vi "Main.vi"(11 "Module Admin":refnum<class "Delacor_lib_QMH_Cloneable Module Admin.lvclass">) -> ()   [LabVIEW 2025, in "Power Supply.lvlib"]
doc: "This template is based off of the Queued Message Handler design pattern and the Queued Message Handler project template that ships with LabVIEW.\n\nThe main difference is that the queue is private to this module and communication between modules is performed via Broadcast and Request events.\n\nRequest events are wrapped in public API methods and are handled in the Event Handling Loop (EHL) of this VI. Any module can register for Broadcast events sent by this module. The EHL generates messages based on user interface actions.\n\nThe Message Handling Loop (MHL) processes messages generated by the EHL, or by other messages. The messages are string values, so new messages can be added easily to the Message Cases case structure in the MHL. Each message cluster can also provide an optional value for Message Data, which is a variant that can be converted to whatever message-specific data is required.\n_____\nBased on DQMH Dev Tools: Project Template 7.1.2.1547."
uses:
  Power Supply.lvlib
  <vilib>/Delacor/Delacor QMH/Libraries/Message Queue_class/Delacor_lib_QMH_Message Queue.lvclass
  Module Data--cluster.ctl
  <vilib>/Utility/miscctls.llb/LVPointTypeDef.ctl
  <vilib>/Delacor/Delacor QMH/Libraries/Message Queue_class/Delacor_lib_QMH_Enqueue Message (Single).vi
  Stop Argument--cluster.ctl
  <vilib>/Delacor/Delacor QMH/Libraries/Cloneable Module Admin_class/Delacor_lib_QMH_Cloneable Module Admin.lvclass
  select child (Reply Payload)--cluster.ctl
  Classes/hardware-selection.ctl
  select child Argument--cluster.ctl
  Classes/generic-power-supply/generic-power-supply.lvclass
  Classes/PSP-603/PSP-603.lvclass
  read config (Reply Payload)--cluster.ctl
  read config Argument--cluster.ctl
  init device (Reply Payload)--cluster.ctl
  init device Argument--cluster.ctl
  close (Reply Payload)--cluster.ctl
  close Argument--cluster.ctl
  output (Reply Payload)--cluster.ctl
  output Argument--cluster.ctl
  set voltage (Reply Payload)--cluster.ctl
  set voltage Argument--cluster.ctl
  set current (Reply Payload)--cluster.ctl
  set current Argument--cluster.ctl
  Controls/Numeric Current.ctl
  read current (Reply Payload)--cluster.ctl
  read current Argument--cluster.ctl
  Controls/Numeric Voltage.ctl
  read voltage (Reply Payload)--cluster.ctl
  read voltage Argument--cluster.ctl
  read state (Reply Payload)--cluster.ctl
  read state Argument--cluster.ctl
  set all outputs (Reply Payload)--cluster.ctl
  set all outputs Argument--cluster.ctl
  C:/Users/grove/Desktop/LabVIEW/Git/atp-station/Libraries/Power Supply/Classes/generic-power-supply/generic-power-supply.lvclass
  C:/Users/grove/Desktop/LabVIEW/Git/atp-station/Libraries/Power Supply/Classes/PSP-603/PSP-603.lvclass
panel:
  out "error out":errorcluster
  out "Status":string
  in  "Simulate EHL Error":bool
  in  "Simulate MHL Error":bool
  # "Other processes communicate with this Module via its Public API (wrappers for its Request Events).\n\nThis Module communicates with other processes via its Broadcast Events.\nAny process that wants to receive these messages can register for this module's Broadcast events."
  # "This template is for the DQMH framework. See the block diagram for more information on how to use this template."
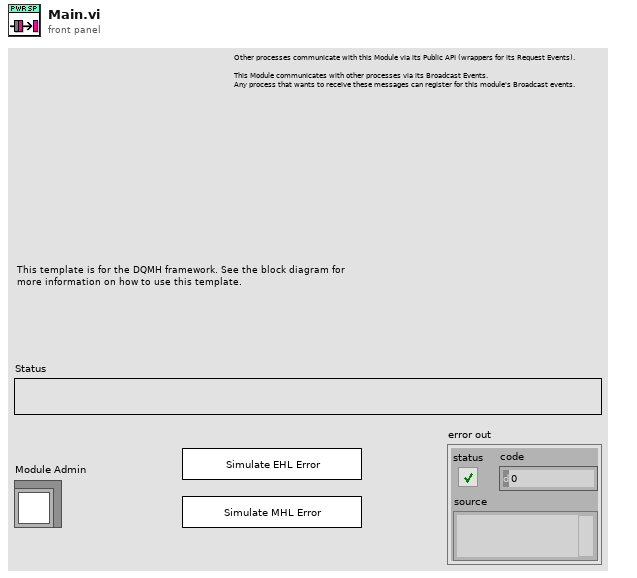
[diagram p1: front panel]
types:
  T1 = typedef "Power Supply.lvlib/Request Events--cluster.ctl" = cluster{"Stop Module":refnum<user-event>, "Show Panel":refnum<user-event>, "Hide Panel":refnum<user-event>, "Show Diagram":refnum<user-event>, "Get Module Execution Status":refnum<user-event>, "select child":refnum<user-event>, "read config":refnum<user-event>, "init device":refnum<user-event>, "close":refnum<user-event>, "output":refnum<user-event>, "set voltage":refnum<user-event>, "set current":refnum<user-event>, "read current":refnum<user-event>, "read voltage":refnum<user-event>, "read state":refnum<user-event>, "set all outputs":refnum<user-event>}
  T2 = typedef "Power Supply.lvlib/Module Data--cluster.ctl" = cluster{"Status":string, "Power Supply Object":refnum<class "generic-power-supply.lvclass">}
  T3 = enum32{"invalid lock state", "Not Locked", "Locked (No Password)", "Password-protected"}
  T4 = typedef "Power Supply.lvlib/Stop Argument--cluster.ctl" = cluster{"Module ID":i32, "Origin":string, "Exit via Stop Module Req?":bool, "Wait for Module to stop?":bool}
  T5 = typedef "Power Supply.lvlib/select child Argument--cluster.ctl" = cluster{"Module ID":i32, "Enum":T6, "Wait Notifier":refnum<notifier>, "wait for reply":bool}
  T6 = typedef "hardware-selection.ctl" = enum16{"Parent", "Simulation", "PSP-603"}
  T7 = typedef "Power Supply.lvlib/read config Argument--cluster.ctl" = cluster{"Module ID":i32, "config json file":path, "Wait Notifier":refnum<notifier>, "wait for reply":bool}
  T8 = typedef "Power Supply.lvlib/init device Argument--cluster.ctl" = cluster{"Module ID":i32, "Variant":variant, "Wait Notifier":refnum<notifier>, "wait for reply":bool}
  T9 = typedef "Power Supply.lvlib/close Argument--cluster.ctl" = cluster{"Module ID":i32, "Wait Notifier":refnum<notifier>, "wait for reply":bool}
  T10 = typedef "Power Supply.lvlib/output Argument--cluster.ctl" = cluster{"Module ID":i32, "Output On/Off":bool, "Wait Notifier":refnum<notifier>, "wait for reply":bool}
  T11 = typedef "Power Supply.lvlib/set voltage Argument--cluster.ctl" = cluster{"Module ID":i32, "Output Voltage":dbl, "Wait Notifier":refnum<notifier>, "wait for reply":bool}
  T12 = typedef "Power Supply.lvlib/set current Argument--cluster.ctl" = cluster{"Module ID":i32, "Output Current":dbl, "Wait Notifier":refnum<notifier>, "wait for reply":bool}
  T13 = typedef "Power Supply.lvlib/read current Argument--cluster.ctl" = cluster{"Module ID":i32, "Wait Notifier":refnum<notifier>, "wait for reply":bool}
  T14 = typedef "Power Supply.lvlib/read voltage Argument--cluster.ctl" = cluster{"Module ID":i32, "Wait Notifier":refnum<notifier>, "wait for reply":bool}
  T15 = typedef "Power Supply.lvlib/read state Argument--cluster.ctl" = cluster{"Module ID":i32, "Wait Notifier":refnum<notifier>, "wait for reply":bool}
  T16 = typedef "Power Supply.lvlib/set all outputs Argument--cluster.ctl" = cluster{"Module ID":i32, "Voltage":dbl, "Current":dbl, "Output On/Off":bool, "Wait Notifier":refnum<notifier>, "wait for reply":bool}
  T17 = typedef "LVPointTypeDef.ctl" = cluster{"Horizontal":i16, "Vertical":i16}
  T18 = enum32{"Invalid", "Standard", "Closed", "Hidden", "Minimized", "Maximized"}
  T19 = typedef "Power Supply.lvlib/select child (Reply Payload)--cluster.ctl" = cluster{"Module ID":i32, "error":errorcluster}
  T20 = typedef "Power Supply.lvlib/read config (Reply Payload)--cluster.ctl" = cluster{"Module ID":i32, "error":errorcluster}
  T21 = typedef "Power Supply.lvlib/init device (Reply Payload)--cluster.ctl" = cluster{"Module ID":i32, "error":errorcluster}
  T22 = typedef "Power Supply.lvlib/close (Reply Payload)--cluster.ctl" = cluster{"Module ID":i32, "error":errorcluster}
  T23 = typedef "Power Supply.lvlib/output (Reply Payload)--cluster.ctl" = cluster{"Module ID":i32, "error":errorcluster}
  T24 = typedef "Power Supply.lvlib/set voltage (Reply Payload)--cluster.ctl" = cluster{"Module ID":i32, "error":errorcluster}
  T25 = typedef "Power Supply.lvlib/set current (Reply Payload)--cluster.ctl" = cluster{"Module ID":i32, "error":errorcluster}
  T26 = typedef "Power Supply.lvlib/read current (Reply Payload)--cluster.ctl" = cluster{"Module ID":i32, "Amps":T27, "error":errorcluster}
  T27 = typedef "Numeric Current.ctl" = dbl
  T28 = typedef "Power Supply.lvlib/read voltage (Reply Payload)--cluster.ctl" = cluster{"Module ID":i32, "Volts":T29, "error":errorcluster}
  T29 = typedef "Numeric Voltage.ctl" = dbl
  T30 = typedef "Power Supply.lvlib/read state (Reply Payload)--cluster.ctl" = cluster{"Module ID":i32, "Variant":variant, "error":errorcluster}
  T31 = typedef "Power Supply.lvlib/set all outputs (Reply Payload)--cluster.ctl" = cluster{"Module ID":i32, "error":errorcluster}
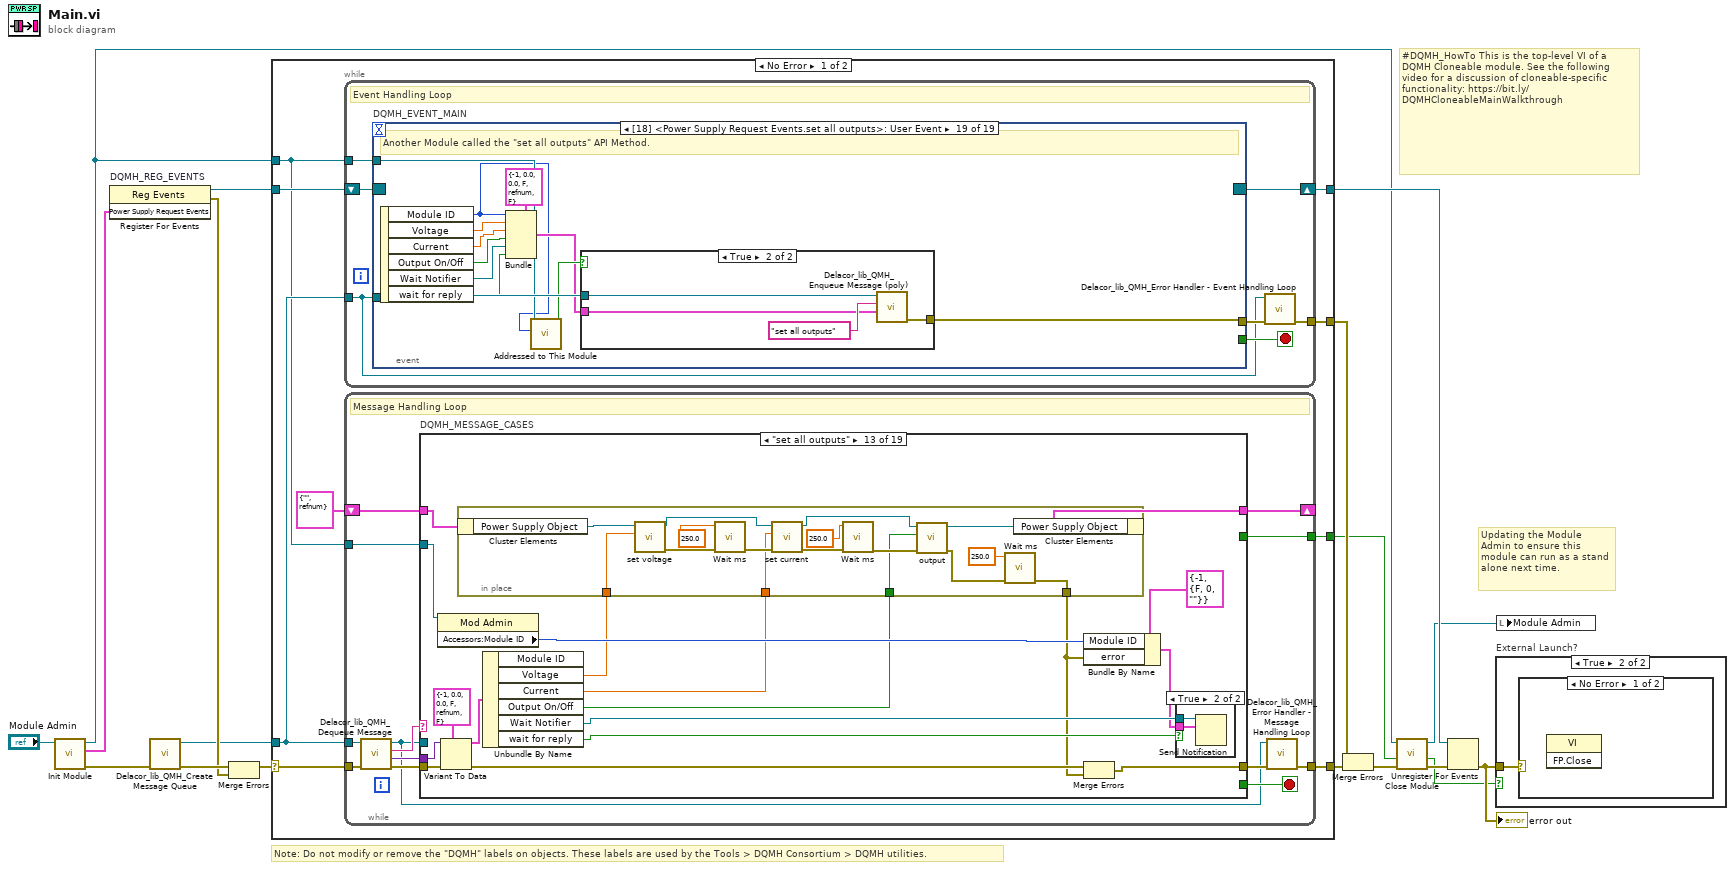
[diagram p0: block diagram]
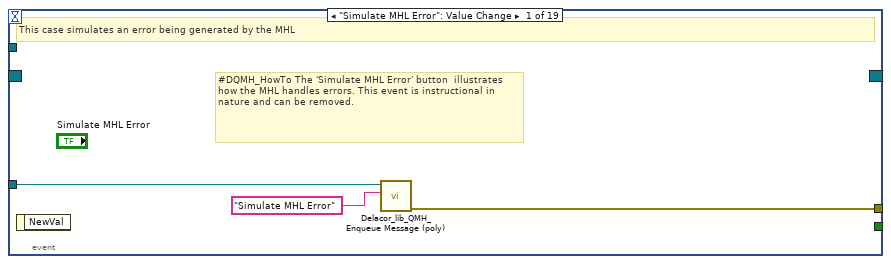
[diagram p2: hidden frame]
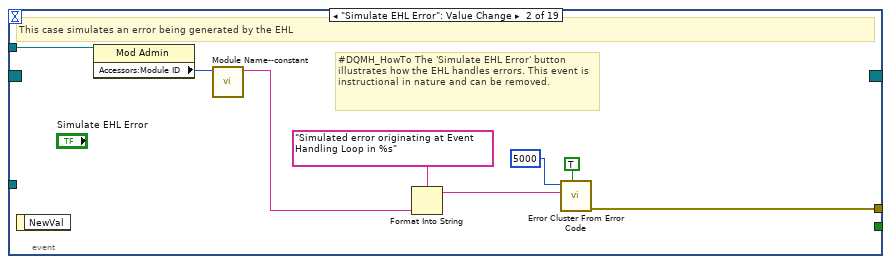
[diagram p3: hidden frame]
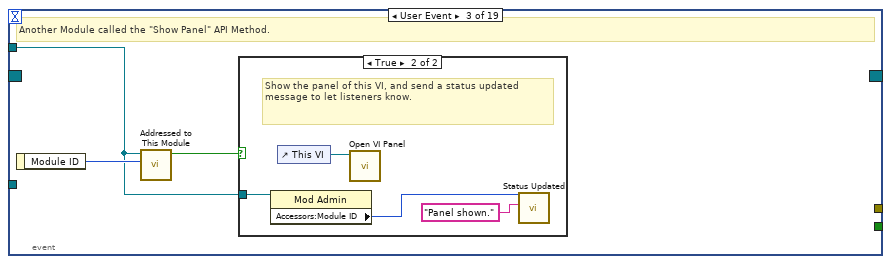
[diagram p4: hidden frame]
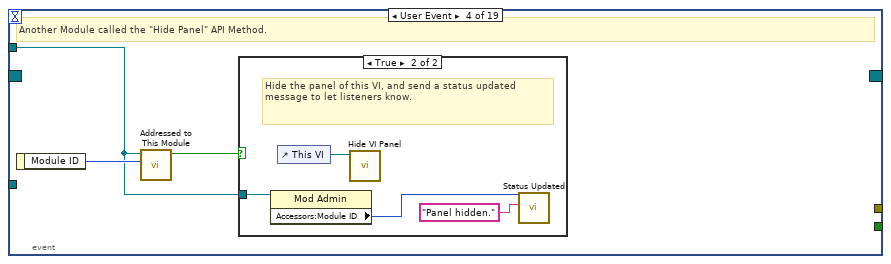
[diagram p6: hidden frame]
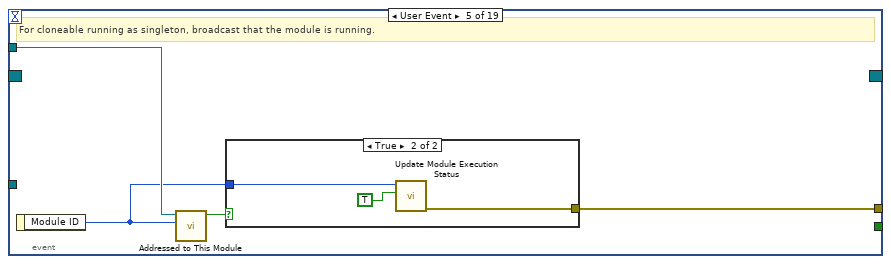
[diagram p8: hidden frame]
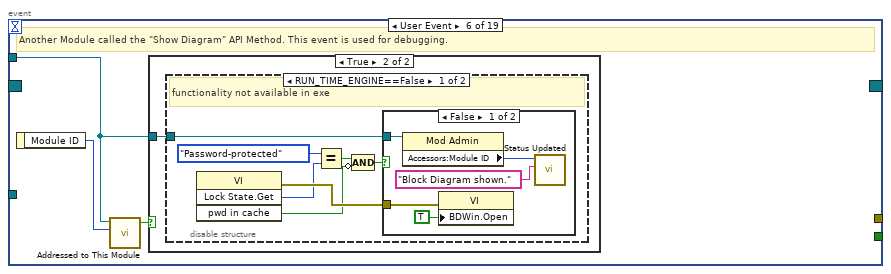
[diagram p10: hidden frame]
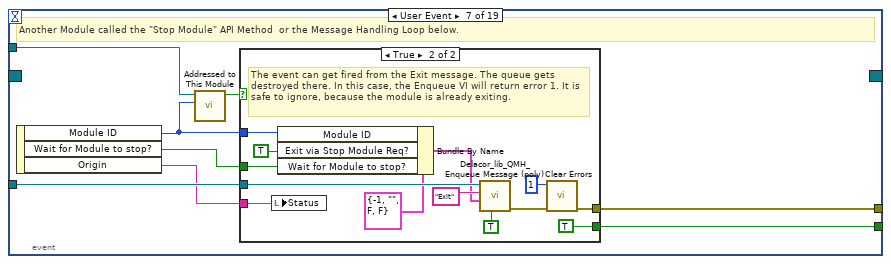
[diagram p14: hidden frame]
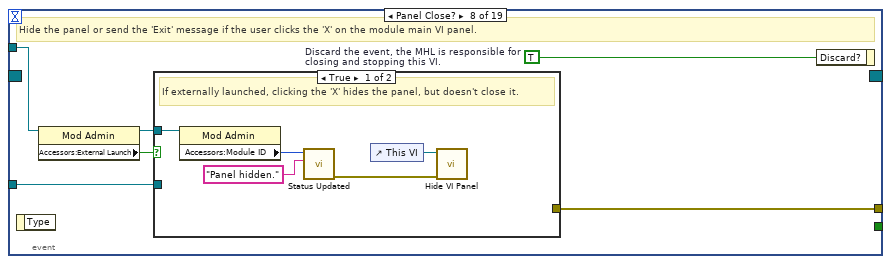
[diagram p16: hidden frame]
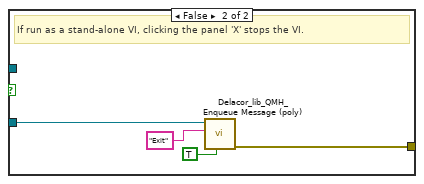
[diagram p17: hidden frame]
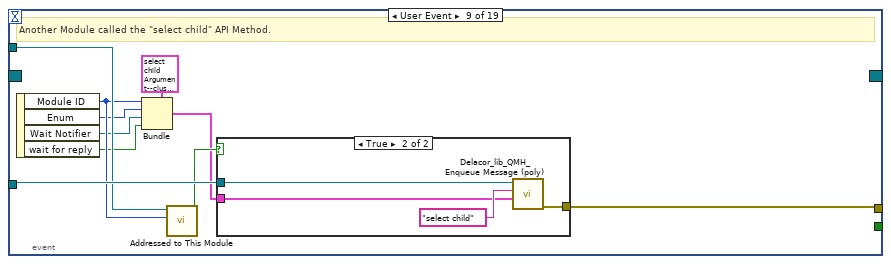
[diagram p18: hidden frame]
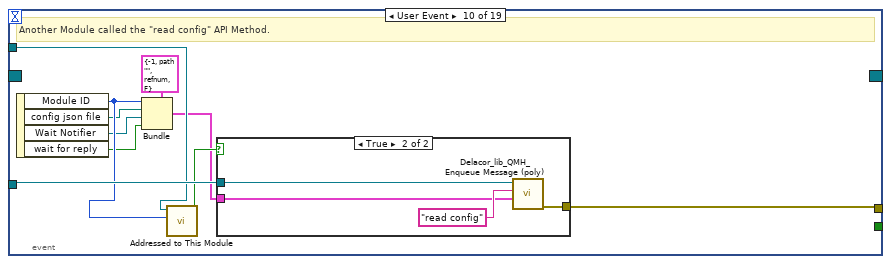
[diagram p20: hidden frame]
diagram:
  # "#DQMH_HowTo This is the top-level VI of a DQMH Cloneable module. See the following video for a discussion of cloneable-specific functionality: https://bit.ly/DQMHCloneableMainWalkthrough"
  # "Note: Do not modify or remove the \"DQMH\" labels on objects. These labels are used by the Tools > DQMH Consortium > DQMH utilities."
  # "Updating the Module Admin to ensure this module can run as a stand alone next time."
  n1 = call "Init Module.vi"("Cloneable Module Admin in"="Module Admin") -> ("error out"=w15:errorcluster, "Power Supply Request Events"=w7:T1, "Cloneable Module Admin out"=w4:refnum<class "Delacor_lib_QMH_Cloneable Module Admin.lvclass">)  [unwired: 8 in]
  n2 = register-events "DQMH_REG_EVENTS"(w7) -> (reference out=w8:refnum<event-registration>, error out=w10:errorcluster)  [unwired: 2 in]
  n3 = call <vilib>:"Delacor_lib_QMH_Create Message Queue.vi"("error in"=w15) -> ("error out"=w12:errorcluster, "Message Queue"=w6:refnum<class "Delacor_lib_QMH_Message Queue.lvclass">)  [unwired: 9 in]
  n4 = Merge Errors(w12, w10) -> (w11:errorcluster)
  n5 = case shown="No Error" w11 {
    selector: w11 -> [w25 w634]
    tunnel: [w27 w633] -> w16
    tunnel: [w24 w632] -> w9
    tunnel: w8 -> [w22 w632]
    tunnel: w6 -> [w21 w625]
    tunnel: [w26 _] -> w17
    tunnel: w4 -> [w20 w628]
    tunnel: [w19 _] -> w2
    frame No Error {
      n6 = while {
        tunnel: w21 -> [w28]
        shift-right: [w31] -> w24
        shift-left: w22 -> [w32]
        tunnel: [w33] -> w26
        tunnel: w20 -> [w29]
        stop <- w30 stop-if-true
        # "Event Handling Loop"
        n7 = event "DQMH_EVENT_MAIN" shown="[18] <Power Supply Request Events.set all outputs>: User Event" {
          selector: w32 -> [_ _ _ _ _ _ _ _ _ _ _ _ _ _ _ _ _ _ _]
          dyn-events: [_ _ _ _ _ _ _ _ _ _ _ _ _ _ _ _ _ _ _] -> w31
          timeout: _ -> [_ _ _ _ _ _ _ _ _ _ _ _ _ _ _ _ _ _ _]
          tunnel: [_ _ _ _ _ _ w86 _ _ _ _ _ _ _ _ _ _ _ _] -> w30
          tunnel: w28 -> [w36 _ _ _ _ _ w89 w106 w128 w142 w156 w169 w183 w197 w211 w224 w237 w250 w266]
          tunnel: [w37 w45 _ _ w63 _ w90 w109 w119 w133 w147 w161 w174 w188 w202 w216 w229 w242 w255] -> w34
          tunnel: w29 -> [_ w44 w46 w53 w61 w67 w88 w107 w126 w140 w154 w167 w181 w195 w209 w222 w235 w248 w264]
          event "Simulate MHL Error": Value Change {
            # "#DQMH_HowTo The 'Simulate MHL Error' button  illustrates how the MHL handles errors. This event is instructional in nature and can be removed."
            # "This case simulates an error being generated by the MHL"
            n8 = event-data() -> ()  [unwired: 1 in, 1 out]
            n9 = call-poly <vilib>:"Delacor_lib_QMH_Enqueue Message (poly).vi"("Message"="Simulate MHL Error", "Message Queue in"=w36) -> ("error out"=w37:errorcluster)  [unwired: 8 in, 1 out]
          }
          event "Simulate EHL Error": Value Change {
            # "#DQMH_HowTo The 'Simulate EHL Error' button  illustrates how the EHL handles errors. This event is instructional in nature and can be removed."
            # "This case simulates an error being generated by the EHL"
            n10 = event-data() -> ()  [unwired: 1 in, 1 out]
            n11 = property on="Property Node" class="Mod Admin"(reference=w44) -> ("Accessors:Module ID"=w43:i32)  [unwired: 1 in, 2 out]
            n12 = call "Module Name--constant.vi"("Module ID"=w43) -> ("Module Name"=w38:string)  [unwired: 10 in]
            n13 = Format Into String(format string="Simulated error originating at Event Handling Loop in %s", w38) -> (resulting string=w41:string)  [unwired: 2 in, 1 out]
            n14 = call <vilib>:"Error Cluster From Error Code.vi"("show call chain? (False)"=TRUE, "error message (\"\")"=w41, "error code (0)"=5000) -> ("error out"=w45:errorcluster)  [unwired: 6 in]
          }
          event User Event {
            # "Another Module called the \"Show Panel\" API Method."
            n15 = event-data() -> ("Module ID"=w47:i32)  [unwired: 1 in]
            n16 = call "Addressed to This Module.vi"("Module ID from Argument"=w47, "Module Admin"=w46) -> ("Addressed to this instance?"=w48:bool)  [unwired: 8 in, 1 out]
            n17 = case shown="True" w48 {
              tunnel: w46 -> [_ w50]
              frame False {
              }
              frame True {
                # "Show the panel of this VI, and send a status updated message to let listeners know."
                n18 = property on="Property Node" class="Mod Admin"(reference=w50) -> ("Accessors:Module ID"=w49:i32)  [unwired: 1 in, 2 out]
                n19 = control-ref of="This VI"() -> (w52:refnum<vi>)
                n20 = call "Open VI Panel.vi"("VI"=w52) -> ()  [unwired: 10 in, 1 out]
                n21 = call "Status Updated.vi"("Status"="Panel shown." ("format string"), "Module ID"=w49) -> ()  [unwired: 9 in, 1 out]
              }
            }
          }
          event User Event {
            # "Another Module called the \"Hide Panel\" API Method."
            n22 = event-data() -> ("Module ID"=w54:i32)  [unwired: 1 in]
            n23 = call "Addressed to This Module.vi"("Module ID from Argument"=w54, "Module Admin"=w53) -> ("Addressed to this instance?"=w55:bool)  [unwired: 8 in, 1 out]
            n24 = case shown="True" w55 {
              tunnel: w53 -> [_ w57]
              frame False {
              }
              frame True {
                # "Hide the panel of this VI, and send a status updated message to let listeners know."
                n25 = property on="Property Node" class="Mod Admin"(reference=w57) -> ("Accessors:Module ID"=w56:i32)  [unwired: 1 in, 2 out]
                n26 = control-ref of="This VI"() -> (w59:refnum<vi>)
                n27 = call "Hide VI Panel.vi"("VI"=w59) -> ()  [unwired: 10 in, 1 out]
                n28 = call "Status Updated.vi"("Status"="Panel hidden." ("format string"), "Module ID"=w56) -> ()  [unwired: 9 in, 1 out]
              }
            }
          }
          event User Event {
            # "For cloneable running as singleton, broadcast that the module is running."
            n29 = event-data() -> ("Module ID"=w60:i32)  [unwired: 1 in]
            n30 = call "Addressed to This Module.vi"("Module ID from Argument"=w60, "Module Admin"=w61) -> ("Addressed to this instance?"=w62:bool)  [unwired: 8 in, 1 out]
            n31 = case shown="True" w62 {
              tunnel: [_ w66] -> w63
              tunnel: w60 -> [_ w65]
              frame False {
              }
              frame True {
                n32 = call "Update Module Execution Status.vi"("Running?"=TRUE, "Module ID"=w65) -> ("error out"=w66:errorcluster)  [unwired: 9 in]
              }
            }
          }
          event User Event {
            # "Another Module called the \"Show Diagram\" API Method. This event is used for debugging."
            n33 = event-data() -> ("Module ID"=w68:i32)  [unwired: 1 in]
            n34 = call "Addressed to This Module.vi"("Module ID from Argument"=w68, "Module Admin"=w67) -> ("Addressed to this instance?"=w69:bool)  [unwired: 8 in, 1 out]
            n35 = case shown="True" w69 {
              tunnel: w67 -> [_ w70]
              frame False {
              }
              frame True {
                n36 = disable-structure shown="RUN_TIME_ENGINE==False" {
                  disable-tunnel: w70 -> [w71 _]
                  frame condition #0 (active) {
                    # "functionality not available in exe"
                    n37 = invoke on="Invoke Node" class="VI" method="Lock State.Get"() -> (error out=w77:errorcluster, "Get Lock State"=w76:T3, "pwd in cache"=w73:bool)  [unwired: 4 in, 1 out]
                    n38 = Equal?(x=T3."Password-protected", y=w76) -> (x = y?=w74:bool)
                    n39 = Compound Arithmetic op=AND(w74, invert w73) -> (w72:bool)
                    n40 = case shown="False" w72 {
                      tunnel: w77 -> [w82 _]
                      tunnel: w71 -> [w79 _]
                      frame False {
                        n41 = property on="Property Node" class="Mod Admin"(reference=w79) -> ("Accessors:Module ID"=w78:i32)  [unwired: 1 in, 2 out]
                        n42 = property on="Property Node" class="VI"(error in=w82, "BDWin.Open"=TRUE ("Block Diagram Window:Open")) -> ()  [unwired: 1 in, 2 out]
                        n43 = call "Status Updated.vi"("Status"="Block Diagram shown." ("format string"), "Module ID"=w78) -> ()  [unwired: 9 in, 1 out]
                      }
                      frame True {
                        # "Password-protected VI, and the password is not in the cache. Do not show the diagram."
                      }
                    }
                  }
                  frame condition #1 {
                  }
                }
              }
            }
          }
          event User Event {
            # "Another Module called the \"Stop Module\" API Method  or the Message Handling Loop below."
            n44 = event-data() -> ("Module ID"=w84:i32, "Wait for Module to stop?"=w85:bool, "Origin"=w83:string)  [unwired: 1 in]
            n45 = call "Addressed to This Module.vi"("Module ID from Argument"=w84, "Module Admin"=w88) -> ("Addressed to this instance?"=w87:bool)  [unwired: 8 in, 1 out]
            n46 = case shown="True" w87 {
              tunnel: [_ w102] -> w90
              tunnel: w89 -> [_ w98]
              tunnel: [_ TRUE] -> w86
              tunnel: w85 -> [_ w93]
              tunnel: w84 -> [_ w95]
              tunnel: w83 -> [_ w91]
              frame False {
              }
              frame True {
                # "The event can get fired from the Exit message. The queue gets destroyed there. In this case, the Enqueue VI will return error 1. It is safe to ignore, because the module is already exiting."
                n47 = local write "Status"(w91) -> ()
                n48 = Bundle By Name(cluster=T4 {"Module ID"=-1, "Origin"="", "Exit via Stop Module Req?"=FALSE, "Wait for Module to stop?"=FALSE} ("Stop Argument"), "Module ID"=w95, "Exit via Stop Module Req?"=TRUE, "Wait for Module to stop?"=w93) -> (w92:T4)
                n49 = call-poly <vilib>:"Delacor_lib_QMH_Enqueue Message (poly).vi"("Priority Message? (F)"=TRUE, "Message Data"=w92, "Message"="Exit", "Message Queue in"=w98) -> ("error out"=w103:errorcluster)  [unwired: 6 in, 1 out]
                n50 = call <vilib>:"Clear Errors.vi"("error in (no error)"=w103, "specific error code to clear (0: all)"=1) -> ("error out"=w102:errorcluster)  [unwired: 4 in, 1 out]
              }
            }
          }
          event Panel Close? {
            w108 = TRUE  # Discard the event, the MHL is responsible for closing and stopping this VI.
            # "Hide the panel or send the 'Exit' message if the user clicks the 'X' on the module main VI panel."
            n51 = event-data() -> ()  [unwired: 1 in, 1 out]
            n52 = property on="Property Node" class="Mod Admin"(reference=w107) -> (reference out=w104:refnum<class "Delacor_lib_QMH_Cloneable Module Admin.lvclass">, "Accessors:External Launch"=w105:bool)  [unwired: 1 in, 1 out]
            n53 = case shown="True" w105 {
              tunnel: w106 -> [_ w117]
              tunnel: [_ w118] -> w109
              tunnel: w104 -> [w112 _]
              frame True {
                # "If externally launched, clicking the 'X' hides the panel, but doesn't close it."
                n54 = property on="Property Node" class="Mod Admin"(reference=w112) -> ("Accessors:Module ID"=w111:i32)  [unwired: 1 in, 2 out]
                n55 = call "Status Updated.vi"("Status"="Panel hidden." ("format string"), "Module ID"=w111) -> ("error out"=w110:errorcluster)  [unwired: 9 in]
                n56 = control-ref of="This VI"() -> (w114:refnum<vi>)
                n57 = call "Hide VI Panel.vi"("error in"=w110, "VI"=w114) -> ()  [unwired: 9 in, 1 out]
              }
              frame False {
                # "If run as a stand-alone VI, clicking the panel 'X' stops the VI."
                n58 = call-poly <vilib>:"Delacor_lib_QMH_Enqueue Message (poly).vi"("Priority Message? (F)"=TRUE, "Message"="Exit", "Message Queue in"=w117) -> ("error out"=w118:errorcluster)  [unwired: 7 in, 1 out]
              }
            }
            n59 = event-data ("Event Filter Node")("Discard?"=w108) -> ()  [unwired: 1 in, 1 out]
          }
          event User Event {
            # "Another Module called the \"select child\" API Method."
            n60 = event-data() -> ("Module ID"=w123:i32, "Enum"=w122:T6, "Wait Notifier"=w121:refnum<notifier>, "wait for reply"=w120:bool)  [unwired: 1 in]
            n61 = Bundle(cluster=T5 {"Module ID"=-1, "Enum"=enum."PSP-603", "Wait Notifier"=refnum, "wait for reply"=FALSE} ("select child Argument"), "Module ID"=w123, "Enum"=w122, "Wait Notifier"=w121, "wait for reply"=w120) -> (w124:T5)
            n62 = call "Addressed to This Module.vi"("Module ID from Argument"=w123, "Module Admin"=w126) -> ("Addressed to this instance?"=w127:bool)  [unwired: 8 in, 1 out]
            n63 = case shown="True" w127 {
              tunnel: w128 -> [_ w132]
              tunnel: w124 -> [_ w130]
              tunnel: [_ w129] -> w119
              frame False {
              }
              frame True {
                n64 = call-poly <vilib>:"Delacor_lib_QMH_Enqueue Message (poly).vi"("Message Data"=w130, "Message"="select child", "Message Queue in"=w132) -> ("error out"=w129:errorcluster)  [unwired: 7 in, 1 out]
              }
            }
          }
          event User Event {
            # "Another Module called the \"read config\" API Method."
            n65 = event-data() -> ("Module ID"=w137:i32, "config json file"=w136:path, "Wait Notifier"=w135:refnum<notifier>, "wait for reply"=w134:bool)  [unwired: 1 in]
            n66 = Bundle(cluster=T7 {"Module ID"=-1, "config json file"=path "", "Wait Notifier"=refnum, "wait for reply"=FALSE} ("read config Argument"), "Module ID"=w137, "config json file"=w136, "Wait Notifier"=w135, "wait for reply"=w134) -> (w138:T7)
            n67 = call "Addressed to This Module.vi"("Module ID from Argument"=w137, "Module Admin"=w140) -> ("Addressed to this instance?"=w141:bool)  [unwired: 8 in, 1 out]
            n68 = case shown="True" w141 {
              tunnel: w142 -> [_ w146]
              tunnel: w138 -> [_ w144]
              tunnel: [_ w143] -> w133
              frame False {
              }
              frame True {
                n69 = call-poly <vilib>:"Delacor_lib_QMH_Enqueue Message (poly).vi"("Message Data"=w144, "Message"="read config", "Message Queue in"=w146) -> ("error out"=w143:errorcluster)  [unwired: 7 in, 1 out]
              }
            }
          }
          event User Event {
            # "Another Module called the \"init device\" API Method."
            n70 = event-data() -> ("Module ID"=w151:i32, "Variant"=w150:variant, "Wait Notifier"=w149:refnum<notifier>, "wait for reply"=w148:bool)  [unwired: 1 in]
            n71 = Bundle(cluster=T8 {"Module ID"=-1, "Variant"=variant, "Wait Notifier"=refnum, "wait for reply"=FALSE} ("init device Argument"), "Module ID"=w151, "Variant"=w150, "Wait Notifier"=w149, "wait for reply"=w148) -> (w152:T8)
            n72 = call "Addressed to This Module.vi"("Module ID from Argument"=w151, "Module Admin"=w154) -> ("Addressed to this instance?"=w155:bool)  [unwired: 8 in, 1 out]
            n73 = case shown="True" w155 {
              tunnel: w156 -> [_ w160]
              tunnel: w152 -> [_ w158]
              tunnel: [_ w157] -> w147
              frame False {
              }
              frame True {
                n74 = call-poly <vilib>:"Delacor_lib_QMH_Enqueue Message (poly).vi"("Message Data"=w158, "Message"="init device", "Message Queue in"=w160) -> ("error out"=w157:errorcluster)  [unwired: 7 in, 1 out]
              }
            }
          }
          event User Event {
            # "Another Module called the \"close\" API Method."
            n75 = event-data() -> ("Module ID"=w164:i32, "Wait Notifier"=w163:refnum<notifier>, "wait for reply"=w162:bool)  [unwired: 1 in]
            n76 = Bundle(cluster=T9 {"Module ID"=-1, "Wait Notifier"=refnum, "wait for reply"=FALSE} ("close Argument"), "Module ID"=w164, "Wait Notifier"=w163, "wait for reply"=w162) -> (w165:T9)
            n77 = call "Addressed to This Module.vi"("Module ID from Argument"=w164, "Module Admin"=w167) -> ("Addressed to this instance?"=w168:bool)  [unwired: 8 in, 1 out]
            n78 = case shown="True" w168 {
              tunnel: w169 -> [_ w173]
              tunnel: w165 -> [_ w171]
              tunnel: [_ w170] -> w161
              frame False {
              }
              frame True {
                n79 = call-poly <vilib>:"Delacor_lib_QMH_Enqueue Message (poly).vi"("Message Data"=w171, "Message"="close", "Message Queue in"=w173) -> ("error out"=w170:errorcluster)  [unwired: 7 in, 1 out]
              }
            }
          }
          event User Event {
            # "Another Module called the \"output\" API Method."
            n80 = event-data() -> ("Module ID"=w178:i32, "Output On/Off"=w177:bool, "Wait Notifier"=w176:refnum<notifier>, "wait for reply"=w175:bool)  [unwired: 1 in]
            n81 = Bundle(cluster=T10 {"Module ID"=-1, "Output On/Off"=FALSE, "Wait Notifier"=refnum, "wait for reply"=FALSE} ("output Argument"), "Module ID"=w178, "Output On/Off"=w177, "Wait Notifier"=w176, "wait for reply"=w175) -> (w179:T10)
            n82 = call "Addressed to This Module.vi"("Module ID from Argument"=w178, "Module Admin"=w181) -> ("Addressed to this instance?"=w182:bool)  [unwired: 8 in, 1 out]
            n83 = case shown="True" w182 {
              tunnel: w183 -> [_ w187]
              tunnel: w179 -> [_ w185]
              tunnel: [_ w184] -> w174
              frame False {
              }
              frame True {
                n84 = call-poly <vilib>:"Delacor_lib_QMH_Enqueue Message (poly).vi"("Message Data"=w185, "Message"="output", "Message Queue in"=w187) -> ("error out"=w184:errorcluster)  [unwired: 7 in, 1 out]
              }
            }
          }
          event User Event {
            # "Another Module called the \"set voltage\" API Method."
            n85 = event-data() -> ("Module ID"=w192:i32, "Output Voltage"=w191:dbl, "Wait Notifier"=w190:refnum<notifier>, "wait for reply"=w189:bool)  [unwired: 1 in]
            n86 = Bundle(cluster=T11 {"Module ID"=-1, "Output Voltage"=10.0, "Wait Notifier"=refnum, "wait for reply"=FALSE} ("set voltage Argument"), "Module ID"=w192, "Output Voltage"=w191, "Wait Notifier"=w190, "wait for reply"=w189) -> (w193:T11)
            n87 = call "Addressed to This Module.vi"("Module ID from Argument"=w192, "Module Admin"=w195) -> ("Addressed to this instance?"=w196:bool)  [unwired: 8 in, 1 out]
            n88 = case shown="True" w196 {
              tunnel: w197 -> [_ w201]
              tunnel: w193 -> [_ w199]
              tunnel: [_ w198] -> w188
              frame False {
              }
              frame True {
                n89 = call-poly <vilib>:"Delacor_lib_QMH_Enqueue Message (poly).vi"("Message Data"=w199, "Message"="set voltage", "Message Queue in"=w201) -> ("error out"=w198:errorcluster)  [unwired: 7 in, 1 out]
              }
            }
          }
          event User Event {
            # "Another Module called the \"set current\" API Method."
            n90 = event-data() -> ("Module ID"=w206:i32, "Output Current"=w205:dbl, "Wait Notifier"=w204:refnum<notifier>, "wait for reply"=w203:bool)  [unwired: 1 in]
            n91 = Bundle(cluster=T12 {"Module ID"=-1, "Output Current"=0.05, "Wait Notifier"=refnum, "wait for reply"=FALSE} ("set current Argument"), "Module ID"=w206, "Output Current"=w205, "Wait Notifier"=w204, "wait for reply"=w203) -> (w207:T12)
            n92 = call "Addressed to This Module.vi"("Module ID from Argument"=w206, "Module Admin"=w209) -> ("Addressed to this instance?"=w210:bool)  [unwired: 8 in, 1 out]
            n93 = case shown="True" w210 {
              tunnel: w211 -> [_ w215]
              tunnel: w207 -> [_ w213]
              tunnel: [_ w212] -> w202
              frame False {
              }
              frame True {
                n94 = call-poly <vilib>:"Delacor_lib_QMH_Enqueue Message (poly).vi"("Message Data"=w213, "Message"="set current", "Message Queue in"=w215) -> ("error out"=w212:errorcluster)  [unwired: 7 in, 1 out]
              }
            }
          }
          event User Event {
            # "Another Module called the \"read current\" API Method."
            n95 = event-data() -> ("Module ID"=w219:i32, "Wait Notifier"=w218:refnum<notifier>, "wait for reply"=w217:bool)  [unwired: 1 in]
            n96 = Bundle(cluster=T13 {"Module ID"=-1, "Wait Notifier"=refnum, "wait for reply"=FALSE} ("read current Argument"), "Module ID"=w219, "Wait Notifier"=w218, "wait for reply"=w217) -> (w220:T13)
            n97 = call "Addressed to This Module.vi"("Module ID from Argument"=w219, "Module Admin"=w222) -> ("Addressed to this instance?"=w223:bool)  [unwired: 8 in, 1 out]
            n98 = case shown="True" w223 {
              tunnel: w224 -> [_ w228]
              tunnel: w220 -> [_ w226]
              tunnel: [_ w225] -> w216
              frame False {
              }
              frame True {
                n99 = call-poly <vilib>:"Delacor_lib_QMH_Enqueue Message (poly).vi"("Message Data"=w226, "Message"="read current", "Message Queue in"=w228) -> ("error out"=w225:errorcluster)  [unwired: 7 in, 1 out]
              }
            }
          }
          event User Event {
            # "Another Module called the \"read voltage\" API Method."
            n100 = event-data() -> ("Module ID"=w232:i32, "Wait Notifier"=w231:refnum<notifier>, "wait for reply"=w230:bool)  [unwired: 1 in]
            n101 = Bundle(cluster=T14 {"Module ID"=-1, "Wait Notifier"=refnum, "wait for reply"=FALSE} ("read voltage Argument"), "Module ID"=w232, "Wait Notifier"=w231, "wait for reply"=w230) -> (w233:T14)
            n102 = call "Addressed to This Module.vi"("Module ID from Argument"=w232, "Module Admin"=w235) -> ("Addressed to this instance?"=w236:bool)  [unwired: 8 in, 1 out]
            n103 = case shown="True" w236 {
              tunnel: w237 -> [_ w241]
              tunnel: w233 -> [_ w239]
              tunnel: [_ w238] -> w229
              frame False {
              }
              frame True {
                n104 = call-poly <vilib>:"Delacor_lib_QMH_Enqueue Message (poly).vi"("Message Data"=w239, "Message"="read voltage", "Message Queue in"=w241) -> ("error out"=w238:errorcluster)  [unwired: 7 in, 1 out]
              }
            }
          }
          event User Event {
            # "Another Module called the \"read state\" API Method."
            n105 = event-data() -> ("Module ID"=w245:i32, "Wait Notifier"=w244:refnum<notifier>, "wait for reply"=w243:bool)  [unwired: 1 in]
            n106 = Bundle(cluster=T15 {"Module ID"=-1, "Wait Notifier"=refnum, "wait for reply"=FALSE} ("read state Argument"), "Module ID"=w245, "Wait Notifier"=w244, "wait for reply"=w243) -> (w246:T15)
            n107 = call "Addressed to This Module.vi"("Module ID from Argument"=w245, "Module Admin"=w248) -> ("Addressed to this instance?"=w249:bool)  [unwired: 8 in, 1 out]
            n108 = case shown="True" w249 {
              tunnel: w250 -> [_ w254]
              tunnel: w246 -> [_ w252]
              tunnel: [_ w251] -> w242
              frame False {
              }
              frame True {
                n109 = call-poly <vilib>:"Delacor_lib_QMH_Enqueue Message (poly).vi"("Message Data"=w252, "Message"="read state", "Message Queue in"=w254) -> ("error out"=w251:errorcluster)  [unwired: 7 in, 1 out]
              }
            }
          }
          event User Event {
            # "Another Module called the \"set all outputs\" API Method."
            n110 = event-data() -> ("Module ID"=w261:i32, "Voltage"=w260:dbl, "Current"=w259:dbl, "Output On/Off"=w258:bool, "Wait Notifier"=w257:refnum<notifier>, "wait for reply"=w256:bool)  [unwired: 1 in]
            n111 = Bundle(cluster=T16 {"Module ID"=-1, "Voltage"=0.0, "Current"=0.0, "Output On/Off"=FALSE, "Wait Notifier"=refnum, "wait for reply"=FALSE} ("set all outputs Argument"), "Module ID"=w261, "Voltage"=w260, "Current"=w259, "Output On/Off"=w258, "Wait Notifier"=w257, "wait for reply"=w256) -> (w262:T16)
            n112 = call "Addressed to This Module.vi"("Module ID from Argument"=w261, "Module Admin"=w264) -> ("Addressed to this instance?"=w265:bool)  [unwired: 8 in, 1 out]
            n113 = case shown="True" w265 {
              tunnel: w266 -> [_ w270]
              tunnel: w262 -> [_ w268]
              tunnel: [_ w267] -> w255
              frame False {
              }
              frame True {
                n114 = call-poly <vilib>:"Delacor_lib_QMH_Enqueue Message (poly).vi"("Message Data"=w268, "Message"="set all outputs", "Message Queue in"=w270) -> ("error out"=w267:errorcluster)  [unwired: 7 in, 1 out]
              }
            }
          }
        }
        n115 = call-dynamic "Delacor_lib_QMH_Error Handler - Event Handling Loop.vi"("error in"=w34, "Message Queue in"=w28) -> ("dup error in"=w33:errorcluster)  [unwired: 8 in, 1 out]
      }
      n116 = while {
        tunnel: w21 -> [w271]
        shift-right: [w278] -> _
        shift-left: T2 {"Status"="", "Power Supply Object"=refnum} ("Data Cluster") -> [w279]
        tunnel: w25 -> [w282]
        tunnel: [w280] -> w27
        tunnel: w20 -> [w273]
        tunnel: [w272] -> w19
        stop <- w277 stop-if-true
        # "Message Handling Loop"
        n117 = call-dynamic "Delacor_lib_QMH_Dequeue Message.vi"("error in"=w282, "Message Queue in"=w271) -> ("error out"=w281:errorcluster, "Message Data"=w275:variant, "Message"=w276:string, "Message Queue out"=w274:refnum<class "Delacor_lib_QMH_Message Queue.lvclass">)  [unwired: 6 in]
        n118 = case "DQMH_MESSAGE_CASES" shown="\"set all outputs\"" w276 {
          selector: w276 -> [_ _ _ _ _ _ _ _ _ _ _ _ _ _ _ _ _ _ w614]
          tunnel: w274 -> [_ _ _ _ _ _ _ _ _ _ _ _ _ _ _ w569 _ w606 _]
          tunnel: w281 -> [w302 w306 w322 w345 w367 w388 w409 w431 w453 w475 w497 w519 w543 w564 w566 w578 w595 w612 w623]
          tunnel: [w300 w306 w313 w336 w358 w379 w400 w422 w444 w466 w488 w510 w534 w563 w566 w574 w594 w607 w624] -> w283
          tunnel: w279 -> [w293 w305 w310 w333 w355 w376 w397 w419 w441 w463 w485 w507 w531 w562 w565 w573 w592 w605 w621]
          tunnel: [w292 w305 w309 w332 w354 w375 w396 w418 w440 w462 w484 w506 w530 w562 w565 w573 w592 w605 w621] -> w278
          tunnel: [_ _ _ _ _ _ _ _ _ _ _ _ _ _ _ _ _ w604 _] -> w277
          tunnel: w275 -> [_ _ w320 w343 w365 w386 w407 w429 w451 w473 w495 w517 w541 _ _ w572 _ w602 _]
          tunnel: w273 -> [w288 _ w311 w334 w356 w377 w398 w420 w442 w464 w486 w508 w532 _ _ w571 w590 w597 w620]
          tunnel: [_ _ _ _ _ _ _ _ _ _ _ _ _ _ _ _ _ w600 _] -> w272
          frame "Initialize" {
            w285 = "Initial Message" ("Initial Message")
            # "#DQMH_CodeNeeded - Initialize the appearance of the front panel."
            # "#DQMH_CodeNeeded - Initialize your state data here."
            # "Initialize - Any operation that needs to be done before the module can receive messages. Synchronize Caller Events.vi will inform Start Module.vi that the module has launched and is ready to receive messages. Module Did Init.vi will broadcast that the module initialized."
            n119 = call "Synchronize Caller Events.vi"("error in"=w302, "Module Admin"=w288) -> ("error out"=w301:errorcluster, "Module Admin out"=w287:refnum<class "Delacor_lib_QMH_Cloneable Module Admin.lvclass">)  [unwired: 8 in]
            n120 = property on="Property Node" class="Mod Admin"(reference=w287) -> ("Accessors:Module ID"=w284:i32, "Accessors:External Launch"=w289:bool)  [unwired: 1 in, 2 out]
            n121 = call "Module Name--constant.vi"("Module ID"=w284) -> ("Module Name"=w297:string)  [unwired: 10 in]
            n122 = property on="Property Node" class="VI"("Front Panel.Title"=w297) -> (reference out=w299:refnum<vi>, error out=w304:errorcluster)  [unwired: 2 in]
            n123 = Select(t=T18."Hidden" ("State"), s=w289, f=T18."Standard" ("State")) -> (s? t:f=w294:T18)
            n124 = invoke on="Invoke Node" class="VI" method="FP.Open"(reference=w299, error in=w304, "State"=w294) -> (reference out=w298:refnum<vi>, error out=w303:errorcluster)  [unwired: 2 in, 3 out]
            n125 = Bundle By Name(cluster=w293, "Status"=w285) -> (w292:T2)
            n126 = invoke on="Invoke Node" class="VI" method="FP.Center"(reference=w298, error in=w303) -> ()  [unwired: 1 in, 3 out]
            n127 = property on="Pane" class="Pane"("Origin"=T17 {"Horizontal"=0, "Vertical"=0}) -> ()  [unwired: 2 in, 2 out]
            n128 = call "Module Name--constant.vi"("Module ID"=w284) -> ("Module Name"=w290:string)  [unwired: 10 in]
            n129 = call "Module Did Init.vi"("error in"=w301, "Initialized?"=TRUE, "Origin"=w290, "Module ID"=w284) -> ("error out"=w300:errorcluster)  [unwired: 7 in]
            "Status" <- w285
          }
          frame "---Module Specific---" {
            # "Separator -- The following cases handle messages specific to this Module."
          }
          frame "select child" {
            w308 = errorcluster {"status"=FALSE, "code"=0, "source"=""} ("error")
            n130 = Variant To Data(error in=w322, type=T5 {"Module ID"=-1, "Enum"=enum."PSP-603", "Wait Notifier"=refnum, "wait for reply"=FALSE} ("select child Argument"), Variant=w320) -> (data=w318:T5, error out=w321:errorcluster)
            n131 = property class="Mod Admin"(reference=w311) -> ("Accessors:Module ID"=w312:i32)  [unwired: 1 in, 2 out]
            n132 = Unbundle By Name(w318) -> ("Enum"=w307:T6, "Wait Notifier"=w317:refnum<notifier>, "wait for reply"=w316:bool)  [unwired: 1 out]
            n133 = in-place {
              in-place-border: w307 -> [w323]
              n134 = in-place-cluster #1(w310) -> ()  [unwired: 1 out]
              n135 = case shown="\"Parent\"" w323 {
                tunnel: [refnum<class "generic-power-supply.lvclass"> refnum ("Power Supply.lvlib:generic-power-supply.lvclass") refnum<class "generic-power-supply.lvclass"> refnum ("Power Supply.lvlib:generic-power-supply.lvclass") refnum<class "PSP-603.lvclass"> refnum ("Power Supply.lvlib:PSP-603.lvclass")] -> w324
                frame "Simulation" {
                }
                frame "Parent" {
                }
                frame "PSP-603" {
                }
              }
              n136 = in-place-cluster #1("Power Supply Object"=w324) -> (w309:T2)
            }
            n137 = Bundle By Name(cluster=T19 {"Module ID"=-1, "error"={"status"=FALSE, "code"=0, "source"=""}} ("select child (Reply Payload)"), "Module ID"=w312, "error"=w308) -> (w315:T19)
            n138 = Merge Errors(w321, w308) -> (w313:errorcluster)
            n139 = case "DQMH_FIRE_NOTIFIER" shown="True" w316 {
              tunnel: w317 -> [_ w329]
              tunnel: w315 -> [_ w328]
              frame False {
              }
              frame True {
                n140 = Send Notification(notification=w328, notifier=w329) -> ()  [unwired: 1 in, 2 out]
              }
            }
          }
          frame "read config" {
            n141 = Variant To Data(error in=w345, type=T7 {"Module ID"=-1, "config json file"=path "", "Wait Notifier"=refnum, "wait for reply"=FALSE} ("read config Argument"), Variant=w343) -> (data=w341:T7, error out=w344:errorcluster)
            n142 = property class="Mod Admin"(reference=w334) -> ("Accessors:Module ID"=w335:i32)  [unwired: 1 in, 2 out]
            n143 = Unbundle By Name(w341) -> ("config json file"=w331:path, "Wait Notifier"=w340:refnum<notifier>, "wait for reply"=w339:bool)  [unwired: 1 out]
            n144 = in-place {
              in-place-border: w331 -> [w347]
              in-place-border: [w346] -> w330
              n145 = in-place-cluster #2(w333) -> ("Power Supply Object"=w349:refnum<class "generic-power-supply.lvclass">)
              n146 = call-dynamic "read config.vi"("File Path"=w347, "generic-power-supply in"=w349) -> ("error out"=w346:errorcluster, "generic-power-supply out"=w348:refnum<class "generic-power-supply.lvclass">)  [unwired: 8 in]
              n147 = in-place-cluster #2("Power Supply Object"=w348) -> (w332:T2)
            }
            n148 = Bundle By Name(cluster=T20 {"Module ID"=-1, "error"={"status"=FALSE, "code"=0, "source"=""}} ("read config (Reply Payload)"), "Module ID"=w335, "error"=w330) -> (w338:T20)
            n149 = Merge Errors(w344, w330) -> (w336:errorcluster)
            n150 = case "DQMH_FIRE_NOTIFIER" shown="True" w339 {
              tunnel: w340 -> [_ w351]
              tunnel: w338 -> [_ w350]
              frame False {
              }
              frame True {
                n151 = Send Notification(notification=w350, notifier=w351) -> ()  [unwired: 1 in, 2 out]
              }
            }
          }
          frame "init device" {
            n152 = Variant To Data(error in=w367, type=T8 {"Module ID"=-1, "Variant"=variant, "Wait Notifier"=refnum, "wait for reply"=FALSE} ("init device Argument"), Variant=w365) -> (data=w363:T8, error out=w366:errorcluster)
            n153 = property class="Mod Admin"(reference=w356) -> ("Accessors:Module ID"=w357:i32)  [unwired: 1 in, 2 out]
            n154 = Unbundle By Name(w363) -> ("Variant"=w352:variant, "Wait Notifier"=w362:refnum<notifier>, "wait for reply"=w361:bool)  [unwired: 1 out]
            n155 = in-place {
              in-place-border: [w369] -> w353
              in-place-border: w352 -> [w368]
              n156 = in-place-cluster #3(w355) -> ("Power Supply Object"=w370:refnum<class "generic-power-supply.lvclass">)
              n157 = call-dynamic "init.vi"("Variant"=w368, "generic-power-supply in"=w370) -> ("error out"=w369:errorcluster, "generic-power-supply out"=w371:refnum<class "generic-power-supply.lvclass">)  [unwired: 8 in]
              n158 = in-place-cluster #3("Power Supply Object"=w371) -> (w354:T2)
            }
            n159 = Bundle By Name(cluster=T21 {"Module ID"=-1, "error"={"status"=FALSE, "code"=0, "source"=""}} ("init device (Reply Payload)"), "Module ID"=w357, "error"=w353) -> (w360:T21)
            n160 = Merge Errors(w366, w353) -> (w358:errorcluster)
            n161 = case "DQMH_FIRE_NOTIFIER" shown="True" w361 {
              tunnel: w362 -> [_ w373]
              tunnel: w360 -> [_ w372]
              frame False {
              }
              frame True {
                n162 = Send Notification(notification=w372, notifier=w373) -> ()  [unwired: 1 in, 2 out]
              }
            }
          }
          frame "close" {
            n163 = Variant To Data(error in=w388, type=T9 {"Module ID"=-1, "Wait Notifier"=refnum, "wait for reply"=FALSE} ("close Argument"), Variant=w386) -> (data=w384:T9, error out=w387:errorcluster)
            n164 = in-place {
              in-place-border: [w389] -> w374
              n165 = in-place-cluster #4(w376) -> ("Power Supply Object"=w391:refnum<class "generic-power-supply.lvclass">)
              n166 = call-dynamic "close.vi"("generic-power-supply in"=w391) -> ("error out"=w389:errorcluster, "generic-power-supply out"=w390:refnum<class "generic-power-supply.lvclass">)  [unwired: 9 in]
              n167 = in-place-cluster #4("Power Supply Object"=w390) -> (w375:T2)
            }
            n168 = property class="Mod Admin"(reference=w377) -> ("Accessors:Module ID"=w378:i32)  [unwired: 1 in, 2 out]
            n169 = Unbundle By Name(w384) -> ("Wait Notifier"=w383:refnum<notifier>, "wait for reply"=w382:bool)  [unwired: 1 out]
            n170 = Bundle By Name(cluster=T22 {"Module ID"=-1, "error"={"status"=FALSE, "code"=0, "source"=""}} ("close (Reply Payload)"), "Module ID"=w378, "error"=w374) -> (w381:T22)
            n171 = Merge Errors(w387, w374) -> (w379:errorcluster)
            n172 = case "DQMH_FIRE_NOTIFIER" shown="True" w382 {
              tunnel: w383 -> [_ w393]
              tunnel: w381 -> [_ w392]
              frame False {
              }
              frame True {
                n173 = Send Notification(notification=w392, notifier=w393) -> ()  [unwired: 1 in, 2 out]
              }
            }
          }
          frame "output" {
            n174 = property class="Mod Admin"(reference=w398) -> ("Accessors:Module ID"=w399:i32)  [unwired: 1 in, 2 out]
            n175 = Variant To Data(error in=w409, type=T10 {"Module ID"=-1, "Output On/Off"=FALSE, "Wait Notifier"=refnum, "wait for reply"=FALSE} ("output Argument"), Variant=w407) -> (data=w405:T10, error out=w408:errorcluster)
            n176 = Unbundle By Name(w405) -> ("Output On/Off"=w395:bool, "Wait Notifier"=w404:refnum<notifier>, "wait for reply"=w403:bool)  [unwired: 1 out]
            n177 = in-place {
              in-place-border: w395 -> [w411]
              in-place-border: [w410] -> w394
              n178 = in-place-cluster #5(w397) -> ("Power Supply Object"=w413:refnum<class "generic-power-supply.lvclass">)
              n179 = call-dynamic "output.vi"("Output [on/off]"=w411, "generic-power-supply in"=w413) -> ("error out"=w410:errorcluster, "generic-power-supply out"=w412:refnum<class "generic-power-supply.lvclass">)  [unwired: 8 in]
              n180 = in-place-cluster #5("Power Supply Object"=w412) -> (w396:T2)
            }
            n181 = Bundle By Name(cluster=T23 {"Module ID"=-1, "error"={"status"=FALSE, "code"=0, "source"=""}} ("output (Reply Payload)"), "Module ID"=w399, "error"=w394) -> (w402:T23)
            n182 = Merge Errors(w408, w394) -> (w400:errorcluster)
            n183 = case "DQMH_FIRE_NOTIFIER" shown="True" w403 {
              tunnel: w404 -> [_ w415]
              tunnel: w402 -> [_ w414]
              frame False {
              }
              frame True {
                n184 = Send Notification(notification=w414, notifier=w415) -> ()  [unwired: 1 in, 2 out]
              }
            }
          }
          frame "set voltage" {
            n185 = Variant To Data(error in=w431, type=T11 {"Module ID"=-1, "Output Voltage"=10.0, "Wait Notifier"=refnum, "wait for reply"=FALSE} ("set voltage Argument"), Variant=w429) -> (data=w427:T11, error out=w430:errorcluster)
            n186 = property class="Mod Admin"(reference=w420) -> ("Accessors:Module ID"=w421:i32)  [unwired: 1 in, 2 out]
            n187 = Unbundle By Name(w427) -> ("Output Voltage"=w417:dbl, "Wait Notifier"=w426:refnum<notifier>, "wait for reply"=w425:bool)  [unwired: 1 out]
            n188 = in-place {
              in-place-border: w417 -> [w433]
              in-place-border: [w432] -> w416
              n189 = in-place-cluster #6(w419) -> ("Power Supply Object"=w435:refnum<class "generic-power-supply.lvclass">)
              n190 = call-dynamic "set voltage.vi"("Voltage"=w433, "generic-power-supply in"=w435) -> ("error out"=w432:errorcluster, "generic-power-supply out"=w434:refnum<class "generic-power-supply.lvclass">)  [unwired: 8 in]
              n191 = in-place-cluster #6("Power Supply Object"=w434) -> (w418:T2)
            }
            n192 = Bundle By Name(cluster=T24 {"Module ID"=-1, "error"={"status"=FALSE, "code"=0, "source"=""}} ("set voltage (Reply Payload)"), "Module ID"=w421, "error"=w416) -> (w424:T24)
            n193 = Merge Errors(w430, w416) -> (w422:errorcluster)
            n194 = case "DQMH_FIRE_NOTIFIER" shown="True" w425 {
              tunnel: w426 -> [_ w437]
              tunnel: w424 -> [_ w436]
              frame False {
              }
              frame True {
                n195 = Send Notification(notification=w436, notifier=w437) -> ()  [unwired: 1 in, 2 out]
              }
            }
          }
          frame "set current" {
            n196 = property class="Mod Admin"(reference=w442) -> ("Accessors:Module ID"=w443:i32)  [unwired: 1 in, 2 out]
            n197 = Variant To Data(error in=w453, type=T12 {"Module ID"=-1, "Output Current"=0.05, "Wait Notifier"=refnum, "wait for reply"=FALSE} ("set current Argument"), Variant=w451) -> (data=w449:T12, error out=w452:errorcluster)
            n198 = Unbundle By Name(w449) -> ("Output Current"=w439:dbl, "Wait Notifier"=w448:refnum<notifier>, "wait for reply"=w447:bool)  [unwired: 1 out]
            n199 = in-place {
              in-place-border: w439 -> [w455]
              in-place-border: [w454] -> w438
              n200 = in-place-cluster #7(w441) -> ("Power Supply Object"=w457:refnum<class "generic-power-supply.lvclass">)
              n201 = call-dynamic "set current.vi"("Current [A]"=w455, "generic-power-supply in"=w457) -> ("error out"=w454:errorcluster, "generic-power-supply out"=w456:refnum<class "generic-power-supply.lvclass">)  [unwired: 8 in]
              n202 = in-place-cluster #7("Power Supply Object"=w456) -> (w440:T2)
            }
            n203 = Bundle By Name(cluster=T25 {"Module ID"=-1, "error"={"status"=FALSE, "code"=0, "source"=""}} ("set current (Reply Payload)"), "Module ID"=w443, "error"=w438) -> (w446:T25)
            n204 = Merge Errors(w452, w438) -> (w444:errorcluster)
            n205 = case "DQMH_FIRE_NOTIFIER" shown="True" w447 {
              tunnel: w448 -> [_ w459]
              tunnel: w446 -> [_ w458]
              frame False {
              }
              frame True {
                n206 = Send Notification(notification=w458, notifier=w459) -> ()  [unwired: 1 in, 2 out]
              }
            }
          }
          frame "read current" {
            n207 = Variant To Data(error in=w475, type=T13 {"Module ID"=-1, "Wait Notifier"=refnum, "wait for reply"=FALSE} ("read current Argument"), Variant=w473) -> (data=w471:T13, error out=w474:errorcluster)
            n208 = property class="Mod Admin"(reference=w464) -> ("Accessors:Module ID"=w465:i32)  [unwired: 1 in, 2 out]
            n209 = in-place {
              in-place-border: [w477] -> w461
              in-place-border: [w476] -> w460
              n210 = in-place-cluster #8(w463) -> ("Power Supply Object"=w479:refnum<class "generic-power-supply.lvclass">)
              n211 = call-dynamic "read current.vi"("generic-power-supply in"=w479) -> ("error out"=w476:errorcluster, "Current [A]"=w477:dbl, "generic-power-supply out"=w478:refnum<class "generic-power-supply.lvclass">)  [unwired: 8 in]
              n212 = in-place-cluster #8("Power Supply Object"=w478) -> (w462:T2)
            }
            n213 = Unbundle By Name(w471) -> ("Wait Notifier"=w470:refnum<notifier>, "wait for reply"=w469:bool)  [unwired: 1 out]
            n214 = Bundle By Name(cluster=T26 {"Module ID"=-1, "Amps"=0.0, "error"={"status"=FALSE, "code"=0, "source"=""}} ("read current (Reply Payload)"), "Module ID"=w465, "Amps"=w461, "error"=w460) -> (w468:T26)
            n215 = Merge Errors(w474, w460) -> (w466:errorcluster)
            n216 = case "DQMH_FIRE_NOTIFIER" shown="True" w469 {
              tunnel: w470 -> [_ w481]
              tunnel: w468 -> [_ w480]
              frame False {
              }
              frame True {
                n217 = Send Notification(notification=w480, notifier=w481) -> ()  [unwired: 1 in, 2 out]
              }
            }
          }
          frame "read voltage" {
            n218 = Variant To Data(error in=w497, type=T14 {"Module ID"=-1, "Wait Notifier"=refnum, "wait for reply"=FALSE} ("read voltage Argument"), Variant=w495) -> (data=w493:T14, error out=w496:errorcluster)
            n219 = in-place {
              in-place-border: [w499] -> w483
              in-place-border: [w498] -> w482
              n220 = in-place-cluster #9(w485) -> ("Power Supply Object"=w501:refnum<class "generic-power-supply.lvclass">)
              n221 = call-dynamic "read voltage.vi"("generic-power-supply in"=w501) -> ("error out"=w498:errorcluster, "Voltage [V]"=w499:dbl, "generic-power-supply out"=w500:refnum<class "generic-power-supply.lvclass">)  [unwired: 8 in]
              n222 = in-place-cluster #9("Power Supply Object"=w500) -> (w484:T2)
            }
            n223 = property class="Mod Admin"(reference=w486) -> ("Accessors:Module ID"=w487:i32)  [unwired: 1 in, 2 out]
            n224 = Unbundle By Name(w493) -> ("Wait Notifier"=w492:refnum<notifier>, "wait for reply"=w491:bool)  [unwired: 1 out]
            n225 = Bundle By Name(cluster=T28 {"Module ID"=-1, "Volts"=0.0, "error"={"status"=FALSE, "code"=0, "source"=""}} ("read voltage (Reply Payload)"), "Module ID"=w487, "Volts"=w483, "error"=w482) -> (w490:T28)
            n226 = Merge Errors(w496, w482) -> (w488:errorcluster)
            n227 = case "DQMH_FIRE_NOTIFIER" shown="True" w491 {
              tunnel: w492 -> [_ w503]
              tunnel: w490 -> [_ w502]
              frame False {
              }
              frame True {
                n228 = Send Notification(notification=w502, notifier=w503) -> ()  [unwired: 1 in, 2 out]
              }
            }
          }
          frame "read state" {
            n229 = Variant To Data(error in=w519, type=T15 {"Module ID"=-1, "Wait Notifier"=refnum, "wait for reply"=FALSE} ("read state Argument"), Variant=w517) -> (data=w515:T15, error out=w518:errorcluster)
            n230 = property class="Mod Admin"(reference=w508) -> ("Accessors:Module ID"=w509:i32)  [unwired: 1 in, 2 out]
            n231 = in-place {
              in-place-border: [w521] -> w505
              in-place-border: [w520] -> w504
              n232 = in-place-cluster #10(w507) -> ("Power Supply Object"=w523:refnum<class "generic-power-supply.lvclass">)
              n233 = call-dynamic "read state.vi"("generic-power-supply in"=w523) -> ("error out"=w520:errorcluster, "Variant"=w521:variant, "generic-power-supply out"=w522:refnum<class "generic-power-supply.lvclass">)  [unwired: 8 in]
              n234 = in-place-cluster #10("Power Supply Object"=w522) -> (w506:T2)
            }
            n235 = Unbundle By Name(w515) -> ("Wait Notifier"=w514:refnum<notifier>, "wait for reply"=w513:bool)  [unwired: 1 out]
            n236 = Bundle By Name(cluster=T30 {"Module ID"=-1, "Variant"=variant, "error"={"status"=FALSE, "code"=0, "source"=""}} ("read state (Reply Payload)"), "Module ID"=w509, "Variant"=w505, "error"=w504) -> (w512:T30)
            n237 = Merge Errors(w518, w504) -> (w510:errorcluster)
            n238 = case "DQMH_FIRE_NOTIFIER" shown="True" w513 {
              tunnel: w514 -> [_ w525]
              tunnel: w512 -> [_ w524]
              frame False {
              }
              frame True {
                n239 = Send Notification(notification=w524, notifier=w525) -> ()  [unwired: 1 in, 2 out]
              }
            }
          }
          frame "set all outputs" {
            n240 = property class="Mod Admin"(reference=w532) -> ("Accessors:Module ID"=w533:i32)  [unwired: 1 in, 2 out]
            n241 = Variant To Data(error in=w543, type=T16 {"Module ID"=-1, "Voltage"=0.0, "Current"=0.0, "Output On/Off"=FALSE, "Wait Notifier"=refnum, "wait for reply"=FALSE} ("set all outputs Argument"), Variant=w541) -> (data=w539:T16, error out=w542:errorcluster)
            n242 = Unbundle By Name(w539) -> ("Voltage"=w529:dbl, "Current"=w528:dbl, "Output On/Off"=w527:bool, "Wait Notifier"=w538:refnum<notifier>, "wait for reply"=w537:bool)  [unwired: 1 out]
            n243 = in-place {
              in-place-border: w529 -> [w558]
              in-place-border: w528 -> [w553]
              in-place-border: w527 -> [w548]
              in-place-border: [w546] -> w526
              n244 = in-place-cluster #11(w531) -> ("Power Supply Object"=w559:refnum<class "generic-power-supply.lvclass">)
              n245 = call-dynamic "set voltage.vi"("Voltage"=w558, "generic-power-supply in"=w559) -> ("error out"=w557:errorcluster, "generic-power-supply out"=w554:refnum<class "generic-power-supply.lvclass">)  [unwired: 8 in]
              n246 = call "Wait ms.vi"("error in (no error)"=w557, "Delay Time (ms)"=250.0) -> ("error out"=w555:errorcluster)  [unwired: 9 in]
              n247 = call-dynamic "set current.vi"("error in (no error)"=w555, "Current [A]"=w553, "generic-power-supply in"=w554) -> ("error out"=w552:errorcluster, "generic-power-supply out"=w550:refnum<class "generic-power-supply.lvclass">)  [unwired: 7 in]
              n248 = call "Wait ms.vi"("error in (no error)"=w552, "Delay Time (ms)"=250.0) -> ("error out"=w549:errorcluster)  [unwired: 9 in]
              n249 = call-dynamic "output.vi"("error in (no error)"=w549, "Output [on/off]"=w548, "generic-power-supply in"=w550) -> ("error out"=w545:errorcluster, "generic-power-supply out"=w547:refnum<class "generic-power-supply.lvclass">)  [unwired: 7 in]
              n250 = call "Wait ms.vi"("error in (no error)"=w545, "Delay Time (ms)"=250.0) -> ("error out"=w546:errorcluster)  [unwired: 9 in]
              n251 = in-place-cluster #11("Power Supply Object"=w547) -> (w530:T2)
            }
            n252 = Bundle By Name(cluster=T31 {"Module ID"=-1, "error"={"status"=FALSE, "code"=0, "source"=""}} ("set all outputs (Reply Payload)"), "Module ID"=w533, "error"=w526) -> (w536:T31)
            n253 = Merge Errors(w542, w526) -> (w534:errorcluster)
            n254 = case "DQMH_FIRE_NOTIFIER" shown="True" w537 {
              tunnel: w538 -> [_ w561]
              tunnel: w536 -> [_ w560]
              frame False {
              }
              frame True {
                n255 = Send Notification(notification=w560, notifier=w561) -> ()  [unwired: 1 in, 2 out]
              }
            }
          }
          frame "---Copy This Frame---" {
            # "Duplicate this frame when creating new messages.  Change this comment in the duplicated frame to describe this message."
            n256 = Merge Errors(w564) -> (w563:errorcluster)
          }
          frame "---Exit and Error Handling---" {
            # "Separator - the following cases handle errors and exit messages."
          }
          frame "Error" {
            # "#DQMH_CodeRecommended - If the module is running in standalone mode (External Launch = FALSE), this code will pop up an error dialog and call the 'Exit' message if an error occurs. Add more fine-grained error management here."
            # "Error - Check the error message data and respond accordingly. This message is sent by the \"Error Handler\" VIs at the end of each loop in this application."
            n257 = property on="Property Node" class="Mod Admin"(reference=w571) -> ("Accessors:External Launch"=w570:bool, "Accessors:Module ID"=w568:i32)  [unwired: 1 in, 2 out]
            n258 = Variant To Data(error in=w578, type=errorcluster {"status"=FALSE, "code"=0, "source"=""} ("error constant"), Variant=w572) -> (data=w567:errorcluster, error out=w576:errorcluster)
            n259 = local write "error out"(w567) -> ()
            n260 = call "Error Reported.vi"("Error"=w567, "Module ID"=w568) -> ()  [unwired: 9 in, 1 out]
            n261 = case shown="False" w570 {
              tunnel: [w583 _] -> w575
              tunnel: w569 -> [w581 _]
              tunnel: w567 -> [w582 _]
              frame False {
                n262 = disable-structure shown="Default" {
                  disable-tunnel: w582 -> [w584 _]
                  frame condition #0 (active) {
                    # "If the module is running standalone, then pop up an error dialog and call the \"Exit\" message."
                    n263 = call <vilib>:"Simple Error Handler.vi"("error in (no error)"=w584) -> ()  [unwired: 4 in, 5 out]
                  }
                  frame condition #1 {
                    # "To prevent the Simple Error Handler VI from being loaded (e.g. when deploying to a Real-Time target), add the Conditional Disable Symbol \"DQMH_Disable_SEH\" to your project and set it to TRUE."
                  }
                }
                n264 = call-poly <vilib>:"Delacor_lib_QMH_Enqueue Message (poly).vi"("Priority Message? (F)"=TRUE, "Message"="Exit", "Message Queue in"=w581) -> ("error out"=w583:errorcluster)  [unwired: 7 in, 1 out]
              }
              frame True {
                # "If the module was launched externally, calling the Error Reported broadcast VI is the only action performed by the \"Error\" message. The module's caller can then process the error appropriately."
              }
            }
            n265 = Merge Errors(w576, w575) -> (w574:errorcluster)
          }
          frame "Simulate MHL Error" {
            # "#DQMH_HowTo The 'Simulate MHL Error' button  illustrates how the MHL handles errors. This event is instructional in nature and can be removed."
            # "Simulate an error occurring at the MHL"
            n266 = property on="Property Node" class="Mod Admin"(reference=w590) -> ("Accessors:Module ID"=w591:i32)  [unwired: 1 in, 2 out]
            n267 = call "Module Name--constant.vi"("Module ID"=w591) -> ("Module Name"=w586:string)  [unwired: 10 in]
            n268 = Format Into String(format string="Simulated error originating at Message Handling Loop in %s", w586) -> (resulting string=w587:string)  [unwired: 2 in, 1 out]
            n269 = call <vilib>:"Error Cluster From Error Code.vi"("show call chain? (False)"=TRUE, "error message (\"\")"=w587, "error code (0)"=5001) -> ("error out"=w593:errorcluster)  [unwired: 6 in]
            n270 = Merge Errors(w595, w593) -> (w594:errorcluster)
          }
          frame "Exit" {
            w603 = 91  # 91: not all Exit messages will have an argument
            w604 = TRUE  # Stop the VI
            # "Release the message queue reference"
            # "#DQMH_CodeNeeded - Add any required cleanup code here."
            # "Exit - Exit the application."
            n271 = Variant To Data(error in=w612, type=T4 {"Module ID"=-1, "Origin"="", "Exit via Stop Module Req?"=FALSE, "Wait for Module to stop?"=FALSE} ("Stop Argument"), Variant=w602) -> (data=w599:T4, error out=w608:errorcluster)
            n272 = call <vilib>:"Clear Errors.vi"("error in (no error)"=w608, "specific error code to clear (0: all)"=w603) -> ("error out"=w611:errorcluster)  [unwired: 4 in, 1 out]
            n273 = property on="Property Node" class="Mod Admin"(reference=w597) -> ("Accessors:Module ID"=w596:i32)  [unwired: 1 in, 2 out]
            n274 = control-ref of="This VI"() -> (w598:refnum<vi>)
            n275 = call-dynamic "Delacor_lib_QMH_Release Message Queue.vi"("error in"=w611, "Message Queue"=w606) -> ("error out"=w610:errorcluster)  [unwired: 9 in]
            n276 = call "Handle Exit.vi"("Stop Argument"=w599, "Module Admin in"=w597, "VI reference"=w598) -> ("error out"=w609:errorcluster, "Wait for Stop?"=w600:bool)  [unwired: 7 in]
            n277 = Merge Errors(w610, w609) -> (w607:errorcluster)
            n278 = call "Error Reported.vi"("Error"=w607, "Module ID"=w596) -> ()  [unwired: 9 in, 1 out]
          }
          frame Default {
            # "'Default' case only runs if there is a message that isn't defined in any of the other cases.  Output a programming error."
            n279 = property on="Property Node" class="Mod Admin"(reference=w620) -> ("Accessors:Module ID"=w619:i32)  [unwired: 1 in, 2 out]
            n280 = call "Module Name--constant.vi"("Module ID"=w619) -> ("Module Name"=w613:string)  [unwired: 10 in]
            n281 = Format Into String(format string="The invalid message string \"%s\" was received in the Message Handling Loop for module \"%s\".", w614, w613) -> (resulting string=w616:string)  [unwired: 2 in, 1 out]
            n282 = call <vilib>:"Error Cluster From Error Code.vi"("show call chain? (False)"=TRUE, "error message (\"\")"=w616, "error code (0)"=1) -> ("error out"=w622:errorcluster)  [unwired: 6 in]
            n283 = Merge Errors(w623, w622) -> (w624:errorcluster)
          }
        }
        n284 = call-dynamic "Delacor_lib_QMH_Error Handler - Message Handling Loop.vi"("error in"=w283, "Message Queue in"=w274) -> ("dup error in"=w280:errorcluster)  [unwired: 8 in, 1 out]
      }
    }
    frame Error {
      n285 = call "Synchronize Caller Events.vi"("Module Admin"=w628) -> ("Module Admin out"=w627:refnum<class "Delacor_lib_QMH_Cloneable Module Admin.lvclass">)  [unwired: 9 in, 1 out]
      n286 = property on="Property Node" class="Mod Admin"(reference=w627) -> ("Accessors:Module ID"=w626:i32)  [unwired: 1 in, 2 out]
      n287 = call-dynamic "Delacor_lib_QMH_Release Message Queue.vi"("error in"=w634, "Message Queue"=w625) -> ("error out"=w633:errorcluster)  [unwired: 9 in]
      n288 = call "Module Name--constant.vi"("Module ID"=w626) -> ("Module Name"=w631:string)  [unwired: 10 in]
      n289 = Format Into String(format string="An error occurred during initialization. %s is no longer running.", w631) -> (resulting string=w629:string)  [unwired: 2 in, 1 out]
      n290 = call "Error Reported.vi"("Additional Information"=w629, "Error"=w633, "Module ID"=w626) -> ()  [unwired: 8 in, 1 out]
    }
  }
  n291 = Merge Errors(w17, w16) -> (w18:errorcluster)
  n292 = call "Close Module.vi"("error in"=w18, "Wait for stop?"=w2, "Module Admin in"=w4) -> ("error out"=w14:errorcluster, "External Launch"=w1:bool, "Module Admin out"=w3:refnum<class "Delacor_lib_QMH_Cloneable Module Admin.lvclass">)  [unwired: 6 in]
  n293 = Unregister For Events(event registration refnum=w9, error in=w14) -> (error out=w13:errorcluster)
  "error out" <- w13
  n294 = case "External Launch?" shown="True" w1 {
    tunnel: w13 -> [_ w635]
    frame False {
    }
    frame True {
      n295 = case shown="No Error" w635 {
        frame No Error {
          n296 = invoke class="VI" method="FP.Close"() -> ()  [unwired: 3 in, 3 out]
        }
        frame Error {
          n297 = disable-structure shown="Default" {
            frame condition #0 (active) {
              n298 = invoke class="VI" method="FP.Open"("Activate"=TRUE ("Activate?")) -> ()  [unwired: 4 in, 5 out]
            }
            frame condition #1 {
              # "Don't show panel on error if running inside a built EXE."
            }
          }
        }
      }
    }
  }
  n299 = local write "Module Admin"(w3) -> ()
